vi "Pusher_Client_Subscribe.vi"(8 "ErrIn":errorcluster, 10 "ChannelName":string, 11 "Client in":refnum<class "Client.lvclass">) -> (0 "ErrOut":errorcluster, 3 "Client out":refnum<class "Client.lvclass">)   [LabVIEW 2009, in "Client.lvclass"]
uses:
  Client.lvclass
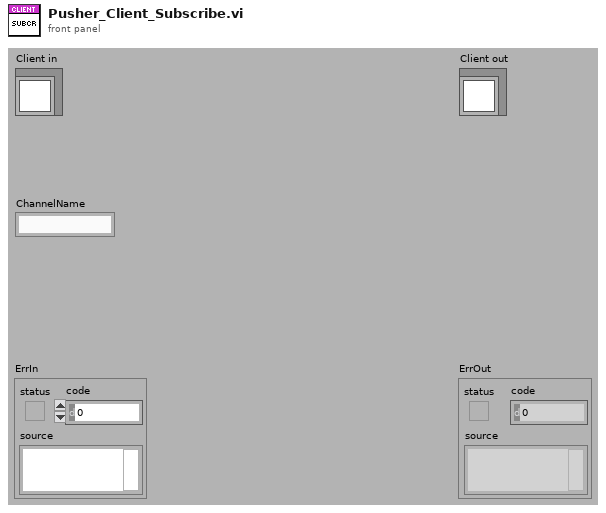
[diagram p1: front panel]
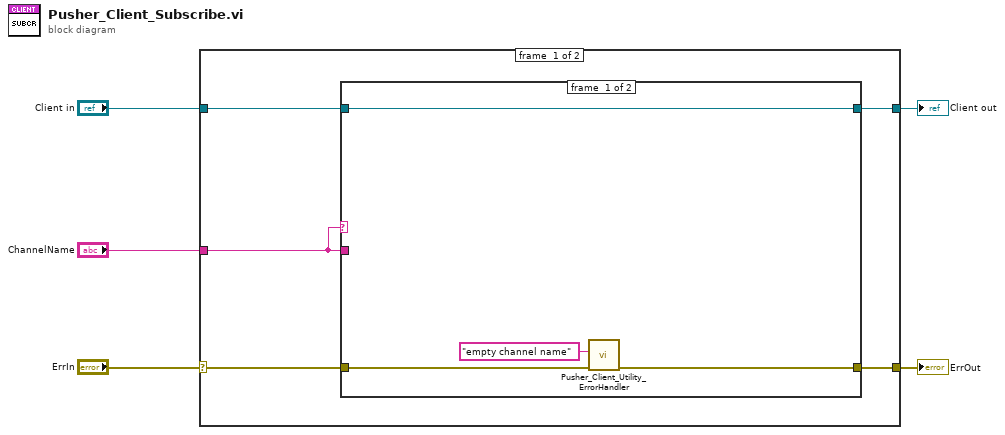
[diagram p0: block diagram]
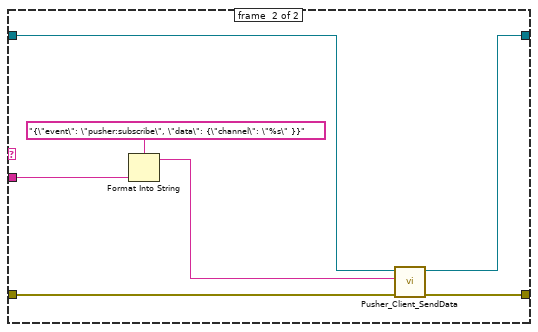
[diagram p2: hidden frame]
diagram:
  n1 = case shown="No Error" "ErrIn" {
    selector: "ErrIn" -> [w10 w23]
    tunnel: [w9 w23] -> w4
    tunnel: [w8 w22] -> w2
    tunnel: "Client in" -> [w7 w22]
    tunnel: "ChannelName" -> [w6 _]
    frame #0 {
      n2 = case shown="\"True\", Default" w6 {
        tunnel: w10 -> [w13 w21]
        tunnel: [w12 w20] -> w9
        tunnel: [w14 w19] -> w8
        tunnel: w6 -> [_ w18]
        tunnel: w7 -> [w14 w15]
        frame #0 {
          n3 = call "Pusher_Client_Utility_ErrorHandler.vi"("ErrIn"=w13, "Additional Message"="empty channel name") -> ("ErrOut"=w12:errorcluster)  [unwired: 9 in]
        }
        frame #1 {
          n4 = Format Into String(format string="{\"event\": \"pusher:subscribe\", \"data\": {\"channel\": \"%s\" }}", w18) -> (resulting string=w16:string)  [unwired: 2 in, 1 out]
          n5 = call "Pusher_Client_SendData.vi"("ErrIn"=w21, "data"=w16, "Client in"=w15) -> ("ErrOut"=w20:errorcluster, "Client out"=w19:refnum<class "Client.lvclass">)  [unwired: 7 in]
        }
      }
    }
    frame #1 {
    }
  }
  "ErrOut" <- w4
  "Client out" <- w2
